vi "Complex Matrix to Compact Array.vi"(2 "matrix type":i32(ring) items=["lower triangular", "upper triangular", "symmetric matrix"], 3 "Matrix A":T1) -> (0 "error":i32, 1 "Compact Array":cluster{"Compact Array":cdb[], "array type":i32} {"array type" items=["lower triangular", "upper triangular", "symmetric matrix"]; "Compact Array" format="%.2f"})   [LabVIEW 2017, in "NI_AALBase.lvlib"]
uses:
  NI_AALBase.lvlib
  ComplexMatrix.ctl
  lvanlys.dll
  NI_Matrix.lvlib
panel:
  # "Complex Matrix to Compact Array"
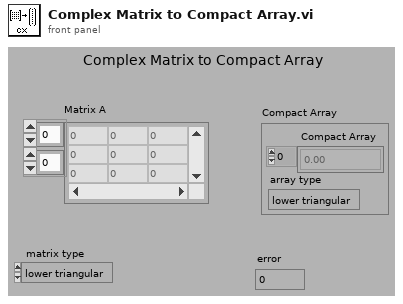
[diagram p1: front panel]
types:
  T1 = typedef "NI_Matrix.lvlib/ComplexMatrix.ctl" = cdb[][]
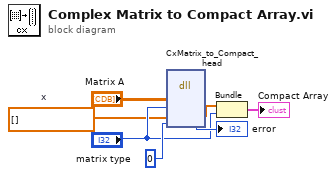
[diagram p0: block diagram]
diagram:
  w2 = cdb[] []  # x
  n1 = dll-call lib="C:/Program Files/National Instruments/LabVIEW 2017/resource/lvanlys.*" fn="CxMatrix_to_Compact_head"("Matrix A"="Matrix A", "matrix type"="matrix type", "x"=w2, 0) -> ("x"=w1:cdb[], →"error":i32)  [unwired: 6 in, 2 out]
  n2 = Bundle("x"=w1, "matrix type"="matrix type") -> (→"Compact Array":cluster{"x":cdb[], "matrix type":i32})  [unwired: 1 in]
